vi "Write Recent User File.vi"(8 "error in (no error)":errorcluster, 10 "recent user file":path, 11 "[P] User in":refnum<class "[P] User.lvclass">) -> (0 "error out":errorcluster, 3 "[P] User out":refnum<class "[P] User.lvclass">)   [LabVIEW 2020, in "[P] User.lvlib" / "[P] User.lvclass"]
uses:
  [P] User.lvclass
  [P] User.lvclass/[P] User.ctl
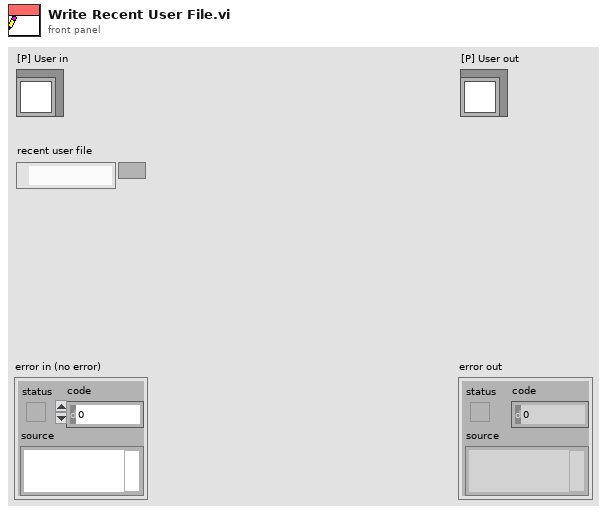
[diagram p1: front panel]
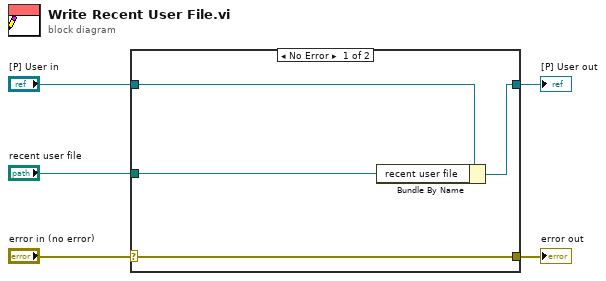
[diagram p0: block diagram]
diagram:
  n1 = case shown="No Error" "error in (no error)" {
    selector: "error in (no error)" -> [w9 w10]
    tunnel: [w9 w10] -> w4
    tunnel: [w7 w11] -> w2
    tunnel: "[P] User in" -> [w8 w11]
    tunnel: "recent user file" -> [w6 _]
    frame No Error {
      n2 = Bundle By Name(cluster=w8, "recent user file"=w6) -> (w7:refnum<class "[P] User.lvclass">)
    }
    frame Error {
    }
  }
  "error out" <- w4
  "[P] User out" <- w2
